vi "CRYTest Input Output Channels Selection.vi"(4 "Record Signal Path In":string[](array[string]), 5 "Output Selected Array":string[][](array[string]), 6 "Play Signal Path In":string[](array[string]), 7 "Acquisition Type":T1(ring), 8 "No.VI":i32, 9 "Play/Record":bool, 10 "Channel Info In":T2[](array[typedef]) {"Coupling" items=["Default"=-1, "RSE"=10083, "NRSE"=10078, "Differential"=10106, "Pseudodifferential"=12529]; "term config" items=["Default"=-1, "RSE"=10083, "NRSE"=10078, "Differential"=10106, "Pseudodifferential"=12529]; "Anti-aliasing Factor (%fs)" format="%.2f"}, 11 "Input Selected Array":string[][](array[string])) -> (1 "Msg Title Str":string, 2 "Message Str":string, 3 "Error Flag":bool)   [LabVIEW 2013]
uses:
  Typedef Control/CRYHardware Channel Info.ctl
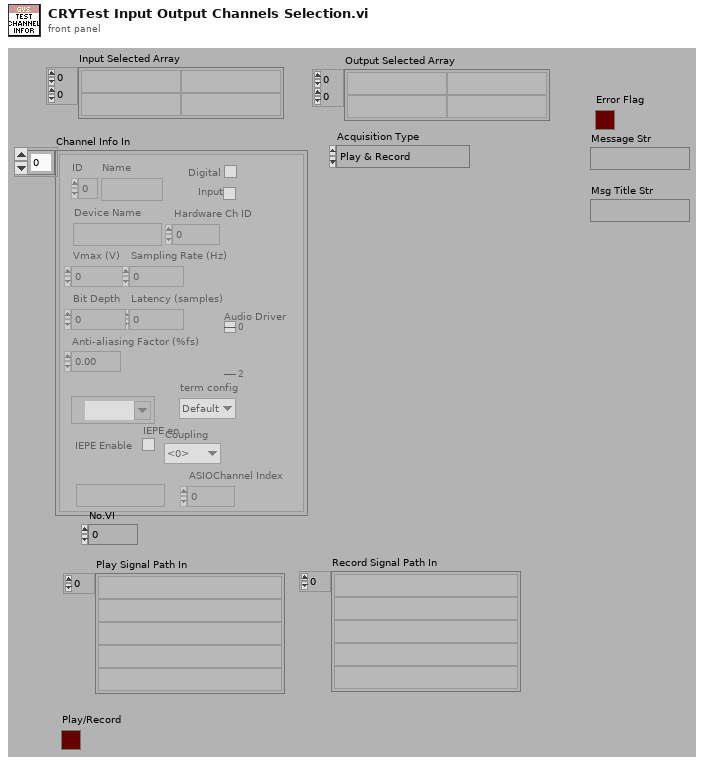
[diagram p1: front panel]
types:
  T1 = enum16{"Play & Record", "Record", "Sine Generator", "Voltmeter", "Oscilloscope", "Spectrum Analyzer", "RTA", "Generator & Voltmeter", "Generator & Oscilloscope", "Generator & Spectrum", "Generator & RTA", "Read From DC Connect"}
  T2 = typedef "CRYHardware Channel Info.ctl" = cluster{"ID":i32, "Name":string, "Digital":bool, "Input":bool, "Device Name":string, "Hardware Ch ID":u8, "Vmax (V)":dbl, "Latency (samples)":dbl, "Sampling Rate (Hz)":u32, "Bit Depth":u32, "Anti-aliasing Factor (%fs)":sgl, "DAQmx Channel":tag, "term config":i32, "Coupling":i32, "IEPE en":bool, "ASIOChannel Name":string, "Audio Driver":u16, "ASIOChannel Index":u8}
  T3 = typedef "CRYWaveform Cluster Array.ctl" = T4[]
  T4 = typedef "CRYWaveform Cluster.ctl" = cluster{"Waveform":cluster{"X0":dbl, "dX":dbl, "Y":sgl[]}, "X data":u16, "Y data":u16, "Y axis":u16, "X unit":string, "Y unit":string, "Y dB ref":dbl, "display Y":bool, "display X":bool, "Overload?":bool, "Test Info":string, "Step No.":i32, "Name":string, "protected":bool, "Sqc history":string[], "Signal Channel ID":i32, "Plot Settings":cluster{"Color":u32, "Interpolation":u8, "Point Style":u8, "Line Style":u8, "Point Color":u32, "Line Width":u8, "Bar Plot Style":u8, "Fill To":i16}, "AutoProtect":bool}
  T5 = typedef "CRYCalibration 2DCluster.ctl" = cluster{"Calibration":T6, "Corr Curve":T7, "EQ Curve":T7, "Sens Curve":T7}
  T6 = typedef "CRYCalibration Cluster.ctl" = cluster{"Calibration Step Name":string, "Device":string, "Correction Curve Name":string, "Equalization Curve Name":string, "Sensitivity Curve Name":string, "Corr Folder and File":string, "EQ Folder and File":string, "Sens Folder and File":string, "Corr Step size":u16, "EQ Step size":u16, "Input":bool, "Last Cal Date (sec)":timestamp, "Cha Name":string, "Corr Curve Found":bool, "EQ Curve Found":bool, "Sens Curve Found":bool, "Signal Type":string, "Calibrated Device":string, "Hz":u32}
  T7 = typedef "CRYData Cluster.ctl" = cluster{"Name":string, "Curve":cluster{"x":dbl, "y":dbl, "z":dbl}[], "X data":u16, "Y data":u16, "Z data":u16, "X axis":u16, "Y axis":u16, "Z axis":u16, "X unit":string, "Y unit":string, "Z unit":string, "X dB ref":dbl, "Y dB ref":dbl, "Z dB ref":dbl, "single val":bool, "protected":bool, "display X":bool, "display Y":bool, "display Z":bool, "Test Info":string, "Step No.":i32, "Plot Settings":cluster{"Color":u32, "Interpolation":u8, "Point Style":u8, "Line Style":u8, "Point Color":u32, "Line Width":u8, "Bar Plot Style":u8, "Fill To":i16}, "AutoProtect":bool}
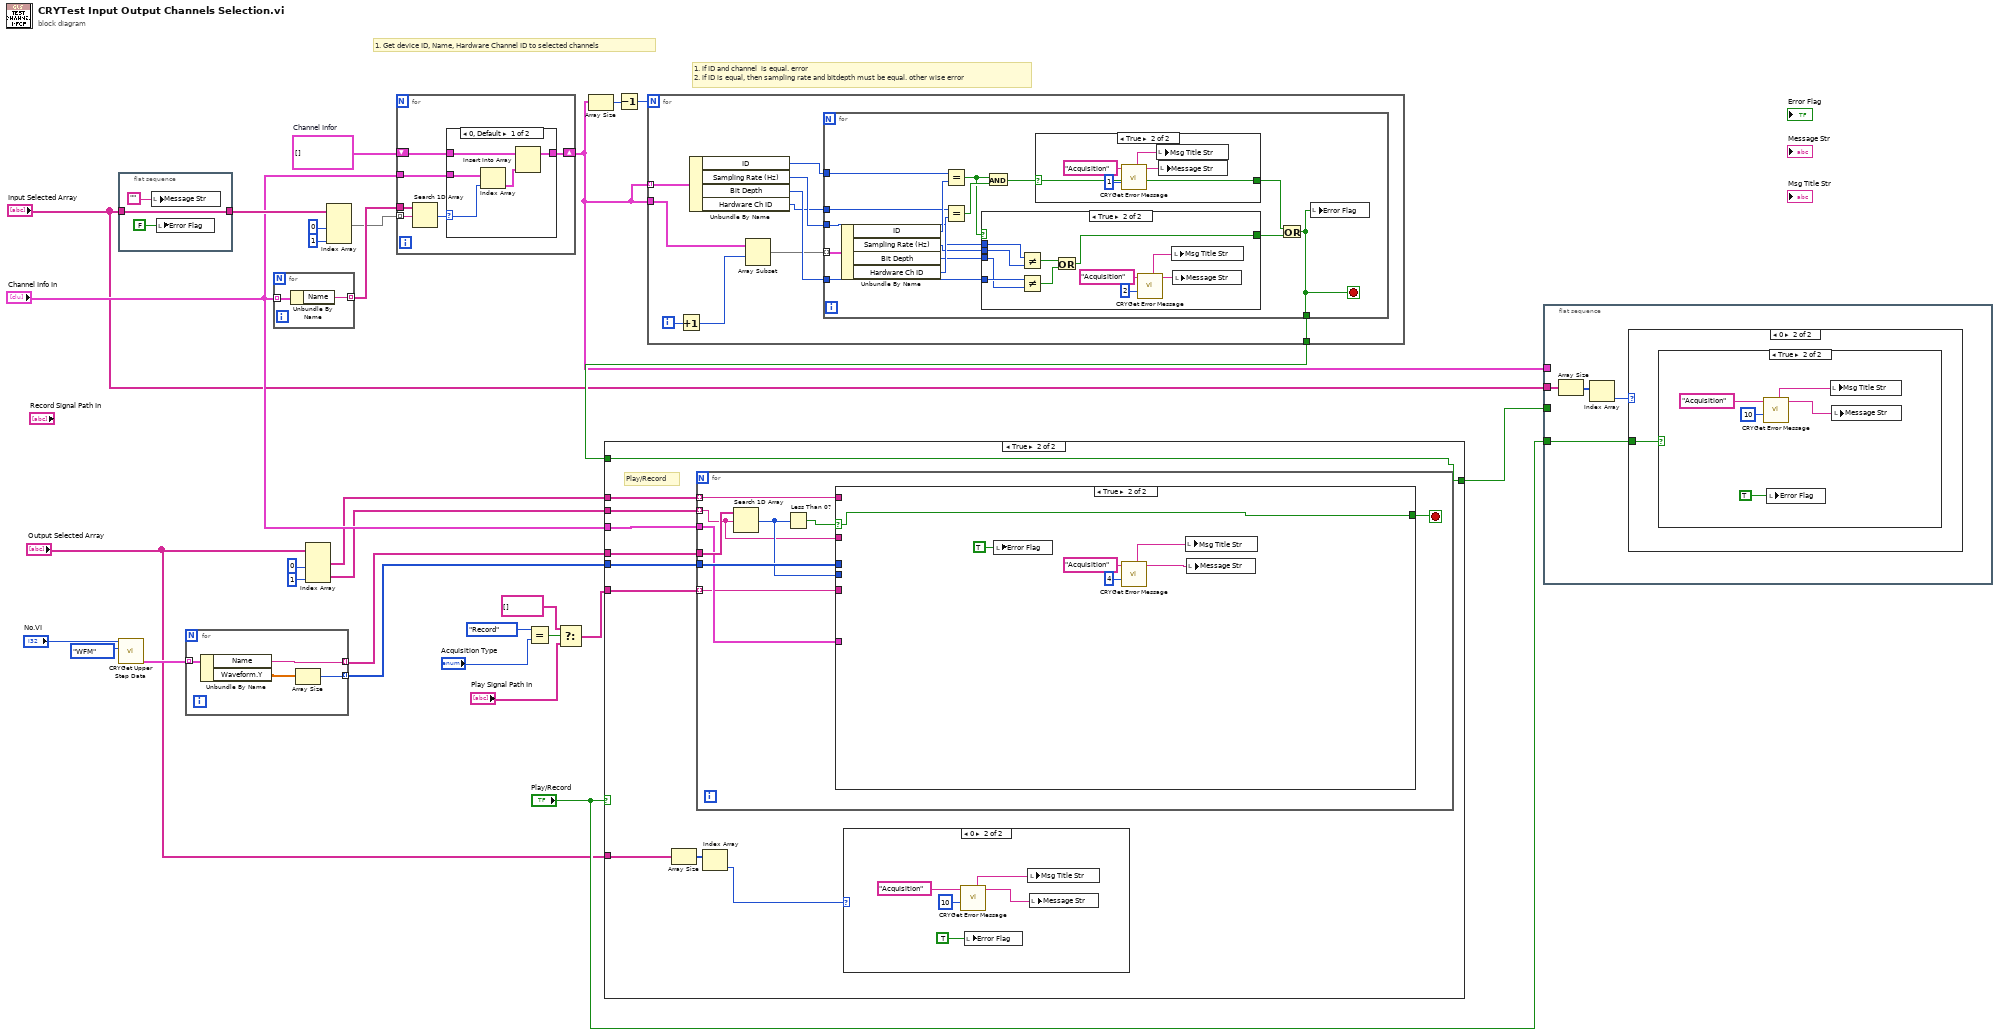
[diagram p0: block diagram]
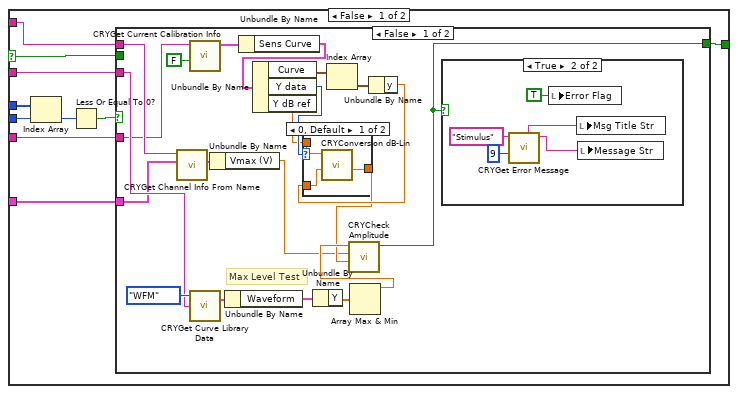
[diagram p6: hidden frame]
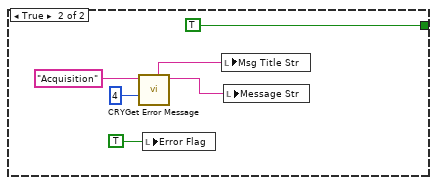
[diagram p9: hidden frame]
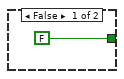
[diagram p11: hidden frame]
diagram:
  w29 = T2[] []  # Channel Infor
  # "1. if ID and channel  is equal. error\n2. if ID is equal, then sampling rate and bitdepth must be equal. other wise error"
  # "1. Get device ID, Name, Hardware Channel ID to selected channels"
  n1 = flat-sequence {
    tunnel: "Input Selected Array" -> [w32]
    tunnel: [w32] -> w25
    frame #0 {
      n2 = local write "Message Str"("" ("Message Str")) -> ()
      n3 = local write "Error Flag"(FALSE ("Error Flag")) -> ()
    }
  }
  n4 = call "CRYGet Upper Step Data.vi"("Type In"=enum16{"Curves", "Values", "Results", "WFM"}."WFM", "No.VI"="No.VI") -> ("Waveform Array"=w20:T3)  [unwired: 9 out]
  n5 = for {
    tunnel: w20 -> [w37] mode=indexing
    tunnel: [w36] -> w19 mode=indexing
    tunnel: [w35] -> w18 mode=indexing
    n6 = Unbundle By Name(w37) -> ("Name"=w36:string, "Waveform.Y"=w34:sgl[])
    n7 = Array Size(array=w34) -> (size(s)=w35:i32)
  }
  n8 = for {
    tunnel: "Channel Info In" -> [w39] mode=indexing
    tunnel: [w38] -> w30 mode=indexing
    n9 = Unbundle By Name(w39) -> ("Name"=w38:string)
  }
  n10 = Index Array(array="Output Selected Array", index (col) #1=0 ("index"), index (col) #2=1 ("index (col)")) -> (element #1=w4:string[], element #2=w3:string[])  [unwired: 2 in]
  n11 = Index Array(array=w25, index (col) #1=0 ("index"), index (col) #2=1 ("index (col)")) -> (element #1=w17:string[])  [unwired: 2 in, 1 out]
  n12 = for {
    tunnel: w17 -> [w43] mode=indexing
    tunnel: w30 -> [w45]
    tunnel: "Channel Info In" -> [w44]
    shift-right: [w41] -> w14
    shift-left: w29 -> [w40]
    n13 = Search 1D Array(1D array=w45, element=w43) -> (index of element=w42:i32)  [unwired: 1 out]
    n14 = case shown="0, Default" w42 {
      selector: w42 -> [w49 _]
      tunnel: w44 -> [w50 _]
      tunnel: [w47 w51] -> w41
      tunnel: w40 -> [w46 w51]
      frame 0, Default {
        n15 = Index Array(array=w50, index=w49) -> (element=w48:T2)
        n16 = Insert Into Array(array=w46, new element=w48) -> (w47:T2[])  [unwired: 1 in]
      }
      frame -1 {
      }
    }
  }
  n17 = Equal?(x=T1."Record" ("Acquisition Type"), y="Acquisition Type") -> (x = y?=w11:bool)
  n18 = Select(t=string[] [] ("Play Signal Path In"), s=w11, f="Play Signal Path In") -> (s? t:f=w8:string[])
  n19 = Array Size(array=w14) -> (size(s)=w27:i32)
  n20 = Decrement(x=w27) -> (x-1=w26:i32)
  n21 = for {
    N: w26 -> [_]
    tunnel: w14 -> [w61] mode=indexing
    tunnel: w14 -> [w56]
    tunnel: [w52] -> w23
    i -> [w60]
    n22 = Increment(x=w60) -> (x+1=w55:i32)
    n23 = Unbundle By Name(w61) -> ("ID"=w59:i32, "Sampling Rate (Hz)"=w58:u32, "Bit Depth"=w57:u32, "Hardware Ch ID"=w53:u8)
    n24 = Array Subset(array=w56, index=w55) -> (w54:T2[])  [unwired: 1 in]
    n25 = for {
      tunnel: w59 -> [w75]
      tunnel: w58 -> [w68]
      tunnel: w57 -> [w67]
      tunnel: w54 -> [w76] mode=indexing
      tunnel: w53 -> [w73]
      tunnel: [w62] -> w52
      stop <- w62 stop-if-true
      n26 = Unbundle By Name(w76) -> ("ID"=w74:i32, "Sampling Rate (Hz)"=w66:u32, "Bit Depth"=w65:u32, "Hardware Ch ID"=w72:u8)
      n27 = Equal?(x=w75, y=w74) -> (x = y?=w70:bool)
      n28 = Equal?(x=w73, y=w72) -> (x = y?=w71:bool)
      n29 = case shown="True" w70 {
        tunnel: [FALSE ("Error Flag") w88] -> w69
        tunnel: w68 -> [_ w94]
        tunnel: w67 -> [_ w92]
        tunnel: w66 -> [_ w93]
        tunnel: w65 -> [_ w91]
        frame False {
        }
        frame True {
          n30 = Not Equal?(x=w94, y=w93) -> (x != y?=w90:bool)
          n31 = Not Equal?(x=w92, y=w91) -> (x != y?=w89:bool)
          n32 = Or(x=w90, y=w89) -> (x .or. y?=w88:bool)
          n33 = call "CRYGet Error Message.vi"("Error No"=2, "Kind"="Acquisition") -> ("Message"=w85:string, "Window Title"=w84:string)  [unwired: 4 in, 4 out]
          n34 = local write "Msg Title Str"(w84) -> ()
          n35 = local write "Message Str"(w85) -> ()
        }
      }
      n36 = And(x=w70, y=w71) -> (x .and. y?=w64:bool)
      n37 = case shown="True" w64 {
        selector: w64 -> [w77 w82]
        tunnel: [w77 w82] -> w63
        frame False {
        }
        frame True {
          n38 = call "CRYGet Error Message.vi"("Error No"=1, "Kind"="Acquisition") -> ("Message"=w79:string, "Window Title"=w78:string)  [unwired: 4 in, 4 out]
          n39 = local write "Msg Title Str"(w78) -> ()
          n40 = local write "Message Str"(w79) -> ()
        }
      }
      n41 = Or(x=w63, y=w69) -> (x .or. y?=w62:bool)
      n42 = local write "Error Flag"(w62) -> ()
    }
  }
  n43 = case shown="True" "Play/Record" {
    tunnel: w3 -> [_ w105]
    tunnel: w23 -> [w95 w99]
    tunnel: w19 -> [_ w104]
    tunnel: w18 -> [_ w103]
    tunnel: w4 -> [_ w102]
    tunnel: "Channel Info In" -> [_ w101]
    tunnel: w8 -> [_ w100]
    tunnel: [w95 w99] -> w15
    tunnel: "Output Selected Array" -> [_ w97]
    frame False {
      # "Record"
    }
    frame True {
      # "Play/Record"
      n44 = Array Size(array=w97) -> (size(s)=w98:i32[])
      n45 = for {
        tunnel: w105 -> [w114] mode=indexing
        tunnel: w104 -> [w118]
        tunnel: w103 -> [w117]
        tunnel: w102 -> [w113] mode=indexing
        tunnel: w101 -> [w112]
        tunnel: w100 -> [w111] mode=indexing
        stop <- w115 stop-if-true
        n46 = Search 1D Array(1D array=w118, element=w114) -> (index of element=w116:i32)  [unwired: 1 out]
        n47 = Less Than 0?(x=w116) -> (x < 0?=w119:bool)
        n48 = case shown="True" w119 {
          selector: w119 -> [w126 w170]
          tunnel: w117 -> [w129 _]
          tunnel: w116 -> [w124 _]
          tunnel: [w125 w170] -> w115
          tunnel: w114 -> [w123 _]
          tunnel: w113 -> [w122 _]
          tunnel: w112 -> [w121 _]
          tunnel: w111 -> [w120 _]
          frame False {
            n49 = Index Array(array=w129, index=w124) -> (element=w128:i32)
            n50 = Less Or Equal To 0?(x=w128) -> (x <= 0?=w127:bool)
            n51 = case shown="False" w127 {
              tunnel: w126 -> [_ _]
              tunnel: [w150 TRUE] -> w125
              tunnel: w123 -> [w135 _]
              tunnel: w122 -> [w134 _]
              tunnel: w121 -> [w133 _]
              tunnel: w120 -> [w130 _]
              frame False {
                # "Max Level Test"
                n52 = call "CRYGet Channel Info From Name.vi"("Channel Info Array In"=w133, "Channel Name"=w134) -> ("ChannelInfo"=w132:T2)  [unwired: 8 in, 1 out]
                n53 = call "CRYGet Current Calibration Info.vi"("Is Input?"=FALSE, "Signal Type Name"=w130) -> ("Calibration All Cluster"=w143:T5)  [unwired: 9 out]
                n54 = call "CRYGet Curve Library Data.vi"("Type"=enum16{"Curves", "Values", "Results", "WFM"}."WFM" ("Type In"), "Data Name"=w135) -> ("Wave"=w148:T4)  [unwired: 4 out]
                n55 = Unbundle By Name(w132) -> ("Vmax (V)"=w131:dbl)
                n56 = Unbundle By Name(w148) -> ("Waveform"=w147:cluster{"X0":dbl, "dX":dbl, "Y":sgl[]})
                n57 = Unbundle By Name(w143) -> ("Sens Curve"=w142:T7)
                n58 = Unbundle By Name(w142) -> ("Curve"=w138:cluster{"x":dbl, "y":dbl, "z":dbl}[], "Y data"=w141:u16, "Y dB ref"=w140:dbl)
                n59 = Unbundle By Name(w147) -> ("Y"=w146:sgl[])
                n60 = Index Array(array=w138) -> (element=w139:cluster{"x":dbl, "y":dbl, "z":dbl})  [unwired: 1 in]
                n61 = Array Max & Min(array=w146) -> (max value=w145:sgl)  [unwired: 3 out]
                n62 = Unbundle By Name(w139) -> ("y"=w137:dbl)
                n63 = case shown="0, Default" w141 {
                  tunnel: w137 -> [w153 w154]
                  tunnel: [w152 w154] -> w136
                  tunnel: w140 -> [w151 _]
                  frame 0, Default {
                    n64 = call "CRYConversion dB-Lin.vi"("dB ref."=w151, "Log In"=w153) -> ("Lin Out"=w152:dbl)  [unwired: 4 in, 3 out]
                  }
                  frame 1 {
                  }
                }
                n65 = call "CRYCheck Amplitude.vi"("Sens Value"=w136, "Vp Out"=w131, "Stimulus max value"=w145) -> ("Overflow"=w150:bool)  [unwired: 8 in]
                n66 = case shown="True" w150 {
                  frame False {
                  }
                  frame True {
                    n67 = call "CRYGet Error Message.vi"("Error No"=9, "Kind"="Stimulus") -> ("Message"=w156:string, "Window Title"=w157:string)  [unwired: 4 in, 4 out]
                    n68 = local write "Error Flag"(TRUE ("Error Flag")) -> ()
                    n69 = local write "Msg Title Str"(w157) -> ()
                    n70 = local write "Message Str"(w156) -> ()
                  }
                }
              }
              frame True {
                n71 = call "CRYGet Error Message.vi"("Error No"=4, "Kind"="Acquisition") -> ("Message"=w161:string, "Window Title"=w160:string)  [unwired: 4 in, 4 out]
                n72 = local write "Error Flag"(TRUE ("Error Flag")) -> ()
                n73 = local write "Msg Title Str"(w160) -> ()
                n74 = local write "Message Str"(w161) -> ()
              }
            }
          }
          frame True {
            n75 = local write "Error Flag"(TRUE ("Error Flag")) -> ()
            n76 = call "CRYGet Error Message.vi"("Error No"=4, "Kind"="Acquisition") -> ("Message"=w167:string, "Window Title"=w166:string)  [unwired: 4 in, 4 out]
            n77 = local write "Msg Title Str"(w166) -> ()
            n78 = local write "Message Str"(w167) -> ()
          }
        }
      }
      n79 = Index Array(array=w98) -> (element=w96:i32)  [unwired: 1 in]
      n80 = case shown="0" w96 {
        frame 1, Default {
        }
        frame 0 {
          n81 = call "CRYGet Error Message.vi"("Error No"=10, "Kind"="Acquisition") -> ("Message"=w108:string, "Window Title"=w107:string)  [unwired: 4 in, 4 out]
          n82 = local write "Error Flag"(TRUE ("Error Flag")) -> ()
          n83 = local write "Msg Title Str"(w107) -> ()
          n84 = local write "Message Str"(w108) -> ()
        }
      }
    }
  }
  n85 = flat-sequence {
    tunnel: w15 -> [_]
    tunnel: w14 -> [_]
    tunnel: "Input Selected Array" -> [w175]
    tunnel: "Play/Record" -> [w172]
    frame #0 {
      n86 = Array Size(array=w175) -> (size(s)=w174:i32[])
      n87 = Index Array(array=w174) -> (element=w173:i32)  [unwired: 1 in]
      n88 = case shown="0" w173 {
        tunnel: w172 -> [_ w176]
        frame 1, Default {
        }
        frame 0 {
          n89 = case shown="True" w176 {
            frame False {
            }
            frame True {
              n90 = call "CRYGet Error Message.vi"("Error No"=10, "Kind"="Acquisition") -> ("Message"=w179:string, "Window Title"=w178:string)  [unwired: 4 in, 4 out]
              n91 = local write "Error Flag"(TRUE ("Error Flag")) -> ()
              n92 = local write "Msg Title Str"(w178) -> ()
              n93 = local write "Message Str"(w179) -> ()
            }
          }
        }
      }
    }
  }
